vi "Procces ICS mode.vi"(8 "error in (no error)":errorcluster, 11 "Simulated_CCD_Camera in":refnum<class "Simulated_CCD_Camera.lvclass">) -> (0 "error out":errorcluster, 3 "Simulated_CCD_Camera out":refnum<class "Simulated_CCD_Camera.lvclass">)   [LabVIEW 2018, in "Simulated_CCD_Camera.lvclass"]
uses:
  Simulated_CCD_Camera.lvclass
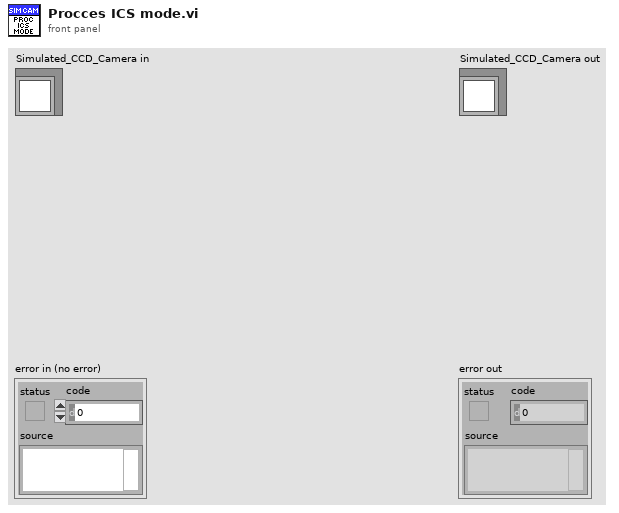
[diagram p1: front panel]
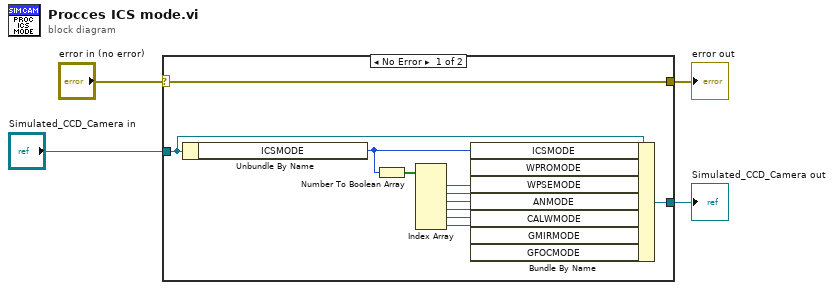
[diagram p0: block diagram]
diagram:
  n1 = case shown="No Error" "error in (no error)" {
    selector: "error in (no error)" -> [w15 w17]
    tunnel: [w15 w17] -> w3
    tunnel: [w13 w16] -> w1
    tunnel: "Simulated_CCD_Camera in" -> [w14 w16]
    frame No Error {
      n2 = Unbundle By Name(w14) -> ("ICSMODE"=w5:u8)
      n3 = Number To Boolean Array(number=w5) -> (Boolean array=w12:bool[])
      n4 = Index Array(array=w12) -> (element #1=w11:bool, element #2=w10:bool, element #3=w9:bool, element #4=w8:bool, element #5=w7:bool, element #6=w6:bool)  [unwired: 6 in]
      n5 = Bundle By Name(cluster=w14, "ICSMODE"=w5, "WPROMODE"=w11, "WPSEMODE"=w10, "ANMODE"=w9, "CALWMODE"=w8, "GMIRMODE"=w7, "GFOCMODE"=w6) -> (w13:refnum<class "Simulated_CCD_Camera.lvclass">)
    }
    frame Error {
    }
  }
  "error out" <- w3
  "Simulated_CCD_Camera out" <- w1
